vi "Double FFT Mesurament (Control - Init Wave&Window - Snapshot - DoubleFFT - Latency - Low Freq) RT Test.vi"() -> ()   [LabVIEW 2014]
uses:
  <vilib>/rvi/interface/nirviOpenFPGA/nirviOpenFPGA.xnode
  <vilib>/rvi/interface/nirviMethod/nirviMethod.xnode
  <vilib>/FPGAPlugInAG/Dynamic/niLvFpga_ConfigureFifo_Dynamic.vi
  <vilib>/rvi/errors/niLvFpgaMergeErrorWithErrorCode.vi
  <vilib>/FPGAPlugInAG/Dynamic/niLvFpga_StartFifo_Dynamic.vi
  <vilib>/FPGAPlugInAG/Dynamic/niLvFpga_Run_Dynamic.vi
  <vilib>/FPGAPlugInAG/Dynamic/niLvFpga_Abort_Dynamic.vi
  <vilib>/rvi/interface/nirviCloseFPGA/nirviCloseFPGA.xnode
  <vilib>/rvi/interface/nirviReadWriteControl/nirviReadWriteControl.xnode
  <vilib>/rvi/interface/Simulation/niFpgaSimulationCallBeginRW.vi
  <vilib>/rvi/errors/niLvFpgaAdjustHostInterfaceError.vi
  <vilib>/FPGAPlugInAG/Dynamic/niLvFpga_ReadFifo_Dynamic.vi
  <vilib>/Platform/TimedLoop/XDataNode/XDataNode.xnode
  <vilib>/Platform/TimedLoop/XDataNode/nitl_modes.ctl
  <vilib>/Platform/TimedLoop/XDataNode/XDNodeRunTimeDep.lvlib
  <vilib>/Platform/TimedLoop/XDataNode/wakeup.ctl
  <vilib>/Platform/TimedLoop/XDataNode/timing_clust.ctl
  <vilib>/FPGAPlugInAG/Dynamic/niLvFpga_Reset_Dynamic.vi
  NiFpgaLv.dll
  <vilib>/Utility/error.llb/Error Cluster From Error Code.vi
  <vilib>/FPGAPlugInAG/Dynamic/niLvFpga_Close_Dynamic.vi
  FPGA Bitfiles/LaserDistanceSen_FPGATarget_DoubleFFTMesuram_744PzgZsl5A.lvbitx
  FPGA Target/Test VIs/Double FFT Mesurament (Control - Init Wave&Window - Snapshot - DoubleFFT - Latency - Low Freq) test.vi
  <vilib>/FPGAPlugInAG/sbRIO-9636/niLvFpga_Open_sbRIO-9636.vi
  <vilib>/rvi/interface/common/dynamic/niFpgaDynamicAddResources.vi
panel:
  in  "stop":bool
  out "maxbin_secondFFT":i32
  out "maxbin_firstFFT":i32
  out "F_rise":dbl
  out "f_fall":dbl
  out "f_mean":dbl
  out "Velocity (m/s)":dbl
  out "Distance (m)":dbl
  in  "Initial Latency points":u32(slide)=10 scale=0.0..1249.0
  out "Second FFT (bin)":dbl[](graph)
  out "Second Signal (points) - Rising Triangular":dbl[](graph)
  out "Elements Remaining FFT":u32
  out "Elements Remaining Signal":u32
  out "First FFT (bin)":dbl[](graph)
  out "First Signal (points) - Falling Triangular":dbl[](graph)
  in  "Snapshot":bool
  in  "Windowing":T1(ring)
  in  "first bin":i32=15
  in  "last bin":i32=255
  in  "lower limit 2":u32(slide)=725 scale=625.0..738.0
  in  "lower limit 1":u32(slide)=100 scale=0.0..113.0
  # "WARNING:\nOnce pressed wait untill the end of operation"
  # "OFFLINE parameters"
  # "Max Detection FFT bin range"
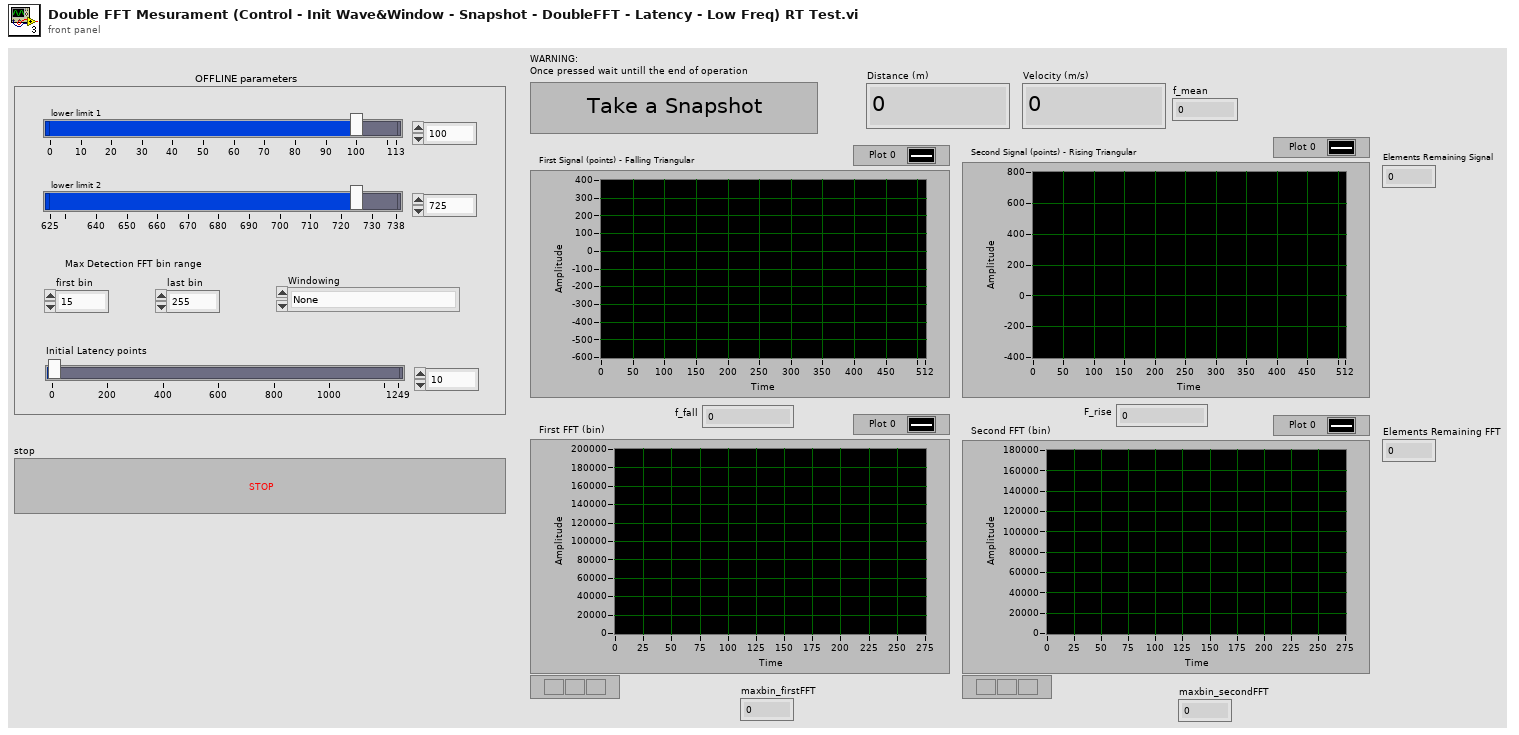
[diagram p1: front panel]
types:
  T1 = enum16{"None", "Hanning", "Hamming", "Blackman", "Blackman-Harris"}
  T2 = typedef "XDNodeRunTimeDep.lvlib/timing_clust.ctl" = cluster{"Expected End [f-1]":u64, "Actual End [f-1]":u64, "Finished Late? [f-1]":bool, "Expected End [i-1]":u64, "Actual End [i-1]":u64, "Finished Late? [i-1]":bool, "Expected Start [i]":u64, "Actual Start [i]":u64, "Expected Start [f]":u64, "Actual Start [f]":u64, "Source Name":string, "Structure Name":string, "Period":i64, "Deadline":i64, "Offset":i64, "Start":i64, "Priority":i32, "Timeout":i32, "Mode":T3, "Wakeup Reason":T4, "Error":errorcluster, "Source Type":string, "Secondary Source Type":string, "Global End Time":u64, "Global Start Time":u64, "Frame Duration":u64, "Iteration Duration":u64, "Assigned CPU":i32, "I/O Scan Engine Mode":u32}
  T3 = typedef "XDNodeRunTimeDep.lvlib/nitl_modes.ctl" = enum32{"No Change", "Process missed periods, maintain original phase", "Discard missed periods, maintain original phase", "Process missed periods, ignore original phase", "Discard missed periods, ignore original phase"}
  T4 = typedef "XDNodeRunTimeDep.lvlib/wakeup.ctl" = enum32{"Normal", "Aborted", "Asynchronous wakeup", "Timing source error", "Timed loop error", "Timeout"}
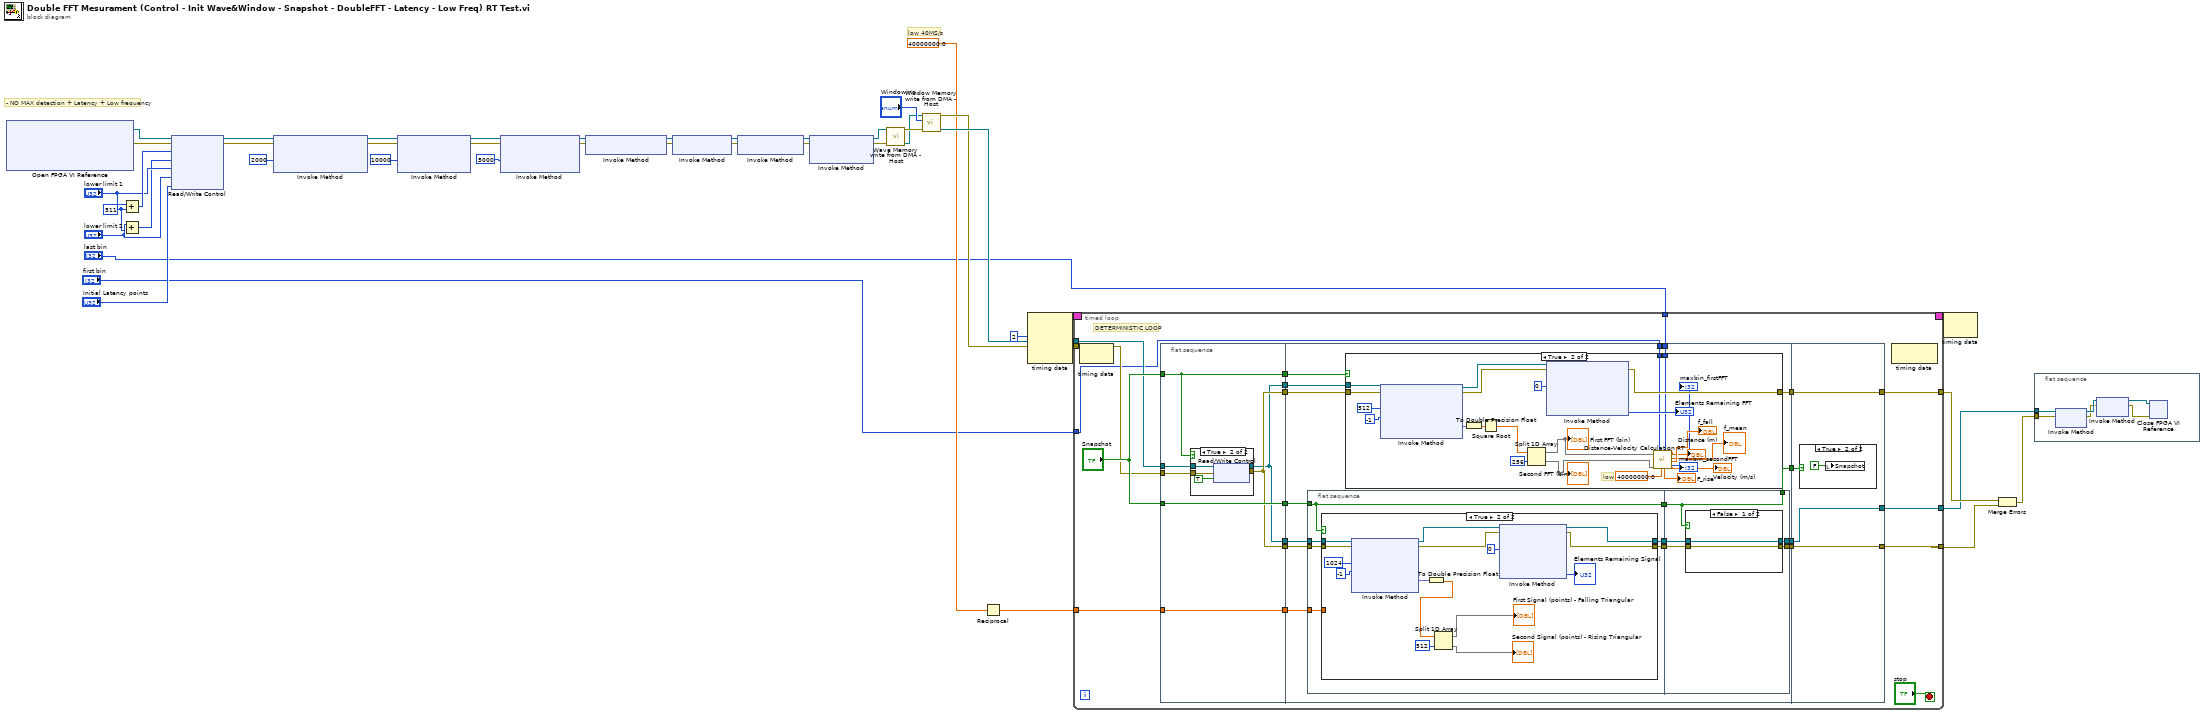
[diagram p0: block diagram]
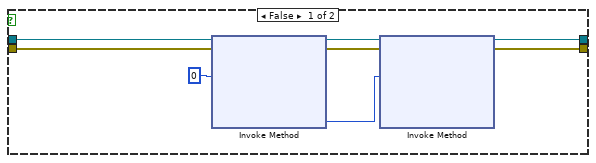
[diagram p3: hidden frame]
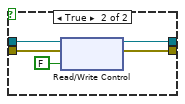
[diagram p4: hidden frame]
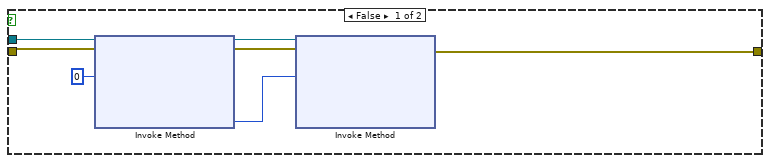
[diagram p5: hidden frame]
diagram:
  w39 = u32 511 ("y")
  # "- NO MAX detection + Latency + Low frequency"
  # "low 40MS/s"
  n1 = xnode "Open FPGA VI Reference"() -> ("FPGA VI Reference Out"=w38:refnum<k20>, "error out"=w37:errorcluster)  [unwired: 2 in]
  n2 = Add(x="lower limit 1", y=w39) -> (x+y=w43:u32)
  n3 = Add(x="lower limit 2", y=w39) -> (x+y=w41:u32)
  n4 = xnode "Read/Write Control"("FPGA VI Reference In"=w38, "error in"=w37, "upper limit 1"=w43, "upper limit 2"=w41, "lower limit 1"="lower limit 1", "lower limit 2"="lower limit 2", "Latency points"="Initial Latency points") -> ("FPGA VI Reference Out"=w33:refnum<k20>, "error out"=w32:errorcluster)
  n5 = xnode "Invoke Method"("FPGA VI Reference In"=w33, "error in"=w32, "Requested Depth"=u32 2000) -> ("FPGA VI Reference Out"=w31:refnum<k20>, "error out"=w30:errorcluster)  [unwired: 1 out]
  n6 = xnode "Invoke Method"("FPGA VI Reference In"=w31, "error in"=w30, "Requested Depth"=u32 10000) -> ("FPGA VI Reference Out"=w29:refnum<k20>, "error out"=w28:errorcluster)  [unwired: 1 out]
  n7 = xnode "Invoke Method"("FPGA VI Reference In"=w29, "error in"=w28, "Requested Depth"=u32 5000) -> ("FPGA VI Reference Out"=w13:refnum<k20>, "error out"=w14:errorcluster)  [unwired: 1 out]
  n8 = xnode "Invoke Method"("FPGA VI Reference In"=w13, "error in"=w14) -> ("FPGA VI Reference Out"=w22:refnum<k20>, "error out"=w21:errorcluster)
  n9 = xnode "Invoke Method"("FPGA VI Reference In"=w22, "error in"=w21) -> ("FPGA VI Reference Out"=w24:refnum<k20>, "error out"=w23:errorcluster)
  n10 = xnode "Invoke Method"("FPGA VI Reference In"=w24, "error in"=w23) -> ("FPGA VI Reference Out"=w11:refnum<k20>, "error out"=w12:errorcluster)
  n11 = xnode "Invoke Method"("FPGA VI Reference In"=w11, "error in"=w12) -> ("FPGA VI Reference Out"=w17:refnum<k20>, "error out"=w16:errorcluster)  [unwired: 1 in]
  n12 = call "Wave Memory write from DMA - Host.vi"("error in"=w16, "FPGA VI Reference In"=w17) -> ("FPGA VI Reference Out"=w2:refnum<k20>, "error out"=w15:errorcluster)  [unwired: 7 in, 1 out]
  n13 = call "Window Memory write from DMA - Host.vi"("error in"=w15, "Enum"="Windowing", "FPGA VI Reference In"=w2) -> ("FPGA VI Reference Out"=w35:refnum<k20>, "error out"=w34:errorcluster)  [unwired: 5 in, 2 out]
  n14 = Reciprocal(x=40000000.0 ("Sample Rate (S/s)")) -> (1/x=w19:dbl)
  n15 = node-c288(i64 2 ("Period")) -> (w10:T2)  [unwired: 3 in]
  n16 = timed-loop {
    tunnel: w35 -> [w59]
    tunnel: w34 -> [w60]
    tunnel: [w62] -> w7
    tunnel: w19 -> [w64]
    tunnel: [w63] -> w6
    timing: w10 -> [_]
    timing-out: [_] -> w9
    tunnel: "first bin" -> [w48]
    tunnel: "last bin" -> [w47]
    tunnel: [w45] -> w1
    stop <- "stop" stop-if-true
    # "DETERMINISTIC LOOP"
    n17 = node-c288() -> ()  [unwired: 1 in, 1 out]
    n18 = flat-sequence {
      tunnel: w59 -> [w69]
      tunnel: w60 -> [w70]
      tunnel: "Snapshot" -> [w67]
      tunnel: "Snapshot" -> [w72]
      tunnel: w64 -> [w73]
      tunnel: [w71] -> w58
      tunnel: [w73] -> w57
      tunnel: [w72] -> w56
      tunnel: [w67] -> w55
      tunnel: [w71] -> w54
      tunnel: [w68] -> w53
      tunnel: [w68] -> w52
      tunnel: w58 -> [w92]
      tunnel: w57 -> [w91]
      tunnel: w56 -> [w85]
      tunnel: w55 -> [w88]
      tunnel: w54 -> [w87]
      tunnel: w53 -> [w86]
      tunnel: w52 -> [w93]
      tunnel: [w90] -> w51
      tunnel: [w89] -> w50
      tunnel: [w84] -> w49
      tunnel: w48 -> [w83]
      tunnel: w47 -> [w82]
      tunnel: [w81] -> w44
      tunnel: [w172] -> w62
      tunnel: [w173] -> w63
      tunnel: w51 -> [w173]
      tunnel: w50 -> [w172]
      tunnel: w49 -> [w171]
      tunnel: [w170] -> w45
      tunnel: w44 -> [w170]
      frame #0 {
        n19 = case shown="True" w67 {
          tunnel: [w74 w79] -> w71
          tunnel: w70 -> [w74 w78]
          tunnel: w69 -> [w75 w77]
          tunnel: [w75 w76] -> w68
          frame False {
          }
          frame True {
            n20 = xnode "Read/Write Control"("FPGA VI Reference In"=w77, "error in"=w78, "snapshot"=TRUE) -> ("FPGA VI Reference Out"=w76:refnum<k20>, "error out"=w79:errorcluster)
          }
        }
      }
      frame #1 {
        n21 = flat-sequence {
          tunnel: w93 -> [w102]
          tunnel: w92 -> [w101]
          tunnel: w91 -> [w100]
          tunnel: w85 -> [w97]
          tunnel: [w99] -> w96
          tunnel: [w98] -> w95
          tunnel: [w97] -> w94
          tunnel: [w128] -> w89
          tunnel: w96 -> [w130]
          tunnel: w95 -> [w129]
          tunnel: w94 -> [w127]
          tunnel: [w127] -> w84
          tunnel: [w126] -> w81
          frame #0 {
            n22 = case shown="True" w97 {
              tunnel: w102 -> [w109 w125]
              tunnel: w101 -> [w107 w124]
              tunnel: [w106 w117] -> w98
              tunnel: w100 -> [_ _]
              tunnel: [w103 w116] -> w99
              frame False {
                n23 = xnode "Invoke Method"("FPGA VI Reference In"=w109, "error in"=w107, "Number of Elements"=u32 0) -> ("FPGA VI Reference Out"=w105:refnum<k20>, "error out"=w104:errorcluster, "Elements Remaining"=w108:u32)  [unwired: 1 in, 1 out]
                n24 = xnode "Invoke Method"("FPGA VI Reference In"=w105, "error in"=w104, "Number of Elements"=w108) -> ("FPGA VI Reference Out"=w103:refnum<k20>, "error out"=w106:errorcluster)  [unwired: 1 in, 2 out]
              }
              frame True {
                n25 = xnode "Invoke Method"("FPGA VI Reference In"=w125, "error in"=w124, "Number of Elements"=u32 1024, "Timeout (ms)"=-1) -> ("FPGA VI Reference Out"=w119:refnum<k20>, "error out"=w118:errorcluster, "Data"=w121:fxp<+/-,12,12>[])  [unwired: 1 out]
                n26 = To Double Precision Float(number=w121) -> (double precision float=w114:dbl[])
                n27 = Split 1D Array(array=w114, index=512) -> (first subarray=→"First Signal (points) - Falling Triangular":dbl[], second subarray=→"Second Signal (points) - Rising Triangular":dbl[])
                n28 = xnode "Invoke Method"("FPGA VI Reference In"=w119, "error in"=w118, "Number of Elements"=u32 0) -> ("FPGA VI Reference Out"=w116:refnum<k20>, "error out"=w117:errorcluster, "Elements Remaining"=→"Elements Remaining Signal":u32)  [unwired: 1 in, 1 out]
              }
            }
          }
          frame #1 {
            n29 = case shown="False" w127 {
              tunnel: [w132 w135] -> w128
              tunnel: w130 -> [w131 w136]
              tunnel: w129 -> [w132 w134]
              tunnel: [w131 w133] -> w126
              frame False {
              }
              frame True {
                n30 = xnode "Read/Write Control"("FPGA VI Reference In"=w136, "error in"=w134, "snapshot"=FALSE) -> ("FPGA VI Reference Out"=w133:refnum<k20>, "error out"=w135:errorcluster)
              }
            }
          }
        }
        n31 = case shown="True" w88 {
          tunnel: w86 -> [w143 w164]
          tunnel: w87 -> [w140 w165]
          tunnel: [w139 w163] -> w90
          tunnel: w83 -> [_ w147]
          tunnel: w82 -> [_ w148]
          frame False {
            n32 = xnode "Invoke Method"("FPGA VI Reference In"=w143, "error in"=w140, "Number of Elements"=u32 0) -> ("FPGA VI Reference Out"=w141:refnum<k20>, "error out"=w138:errorcluster, "Elements Remaining"=w142:u32)  [unwired: 1 in, 1 out]
            n33 = xnode "Invoke Method"("FPGA VI Reference In"=w141, "error in"=w138, "Number of Elements"=w142) -> ("error out"=w139:errorcluster)  [unwired: 1 in, 3 out]
          }
          frame True {
            # "low"
            n34 = xnode "Invoke Method"("FPGA VI Reference In"=w164, "error in"=w165, "Number of Elements"=u32 512, "Timeout (ms)"=-1) -> ("FPGA VI Reference Out"=w161:refnum<k20>, "error out"=w162:errorcluster, "Data"=w167:fxp<+,44,44>[])  [unwired: 1 out]
            n35 = To Double Precision Float(number=w167) -> (double precision float=w166:dbl[])
            n36 = Square Root(x=w166) -> (sqrt(x)=w158:dbl[])
            n37 = Split 1D Array(array=w158, index=256) -> (first subarray=w156:dbl[], second subarray=w155:dbl[])
            "First FFT (bin)" <- w156
            "Second FFT (bin)" <- w155
            n38 = xnode "Invoke Method"("FPGA VI Reference In"=w161, "error in"=w162, "Number of Elements"=u32 0) -> ("error out"=w163:errorcluster, "Elements Remaining"=→"Elements Remaining FFT":u32)  [unwired: 1 in, 2 out]
            n39 = call "Distance-Velocity Calculation RT.vi"("First FFT"=w156, "Second FFT"=w155, "first FFT bin"=w147, "Sample Rate (S/s)"=40000000.0, "last FFT bin"=w148) -> ("F_rise"=→"F_rise":dbl, "maxbin_firstFFT"=→"maxbin_firstFFT":i32, "maxbin_secondFFT"=→"maxbin_secondFFT":i32, "Distance (m)"=→"Distance (m)":dbl, "f_mean"=→"f_mean":dbl, "F_fall"=→"f_fall":dbl, "Velocity (m/s)"=→"Velocity (m/s)":dbl)  [unwired: 8 in]
          }
        }
      }
      frame #2 {
        n40 = case shown="True" w171 {
          frame False {
          }
          frame True {
            n41 = local write "Snapshot"(FALSE ("Snapshot")) -> ()
          }
        }
      }
    }
    n42 = node-c288() -> ()  [unwired: 1 in, 1 out]
  }
  n43 = node-c288(w9) -> ()  [unwired: 1 out]
  n44 = Merge Errors(w6, w7) -> (w20:errorcluster)
  n45 = flat-sequence {
    tunnel: w20 -> [w180]
    tunnel: w1 -> [w175]
    frame #0 {
      n46 = xnode "Invoke Method"("FPGA VI Reference In"=w175, "error in"=w180) -> ("FPGA VI Reference Out"=w177:refnum<k20>, "error out"=w176:errorcluster)
      n47 = xnode "Invoke Method"("FPGA VI Reference In"=w177, "error in"=w176) -> ("FPGA VI Reference Out"=w178:refnum<k20>, "error out"=w179:errorcluster)
      n48 = xnode "Close FPGA VI Reference"("FPGA VI Reference In"=w178, "error in"=w179) -> ()  [unwired: 1 out]
    }
  }
